vi "Dashboard Main.vi"() -> ()   [LabVIEW 2014]
uses:
  <vilib>/event_ctls.llb/eventvkey.ctl
  <vilib>/Rock Robotics/WPI/Dashboard/WPI_DashboardLogging Global.vi
  <vilib>/Rock Robotics/Network Tables/SD Read Number.vi
  <vilib>/Utility/config.llb/Write Key (String).vi
  <vilib>/Utility/config.llb/Write Key (I32).vi
  <vilib>/Rock Robotics/Network Tables/SD Write Numeric Array.vi
  <vilib>/Utility/config.llb/NI_LVConfig.lvlib
panel:
  out "Numeric":u32
  in  "TCP":refnum<k5>
  in  "Rec Mode":enum32{"Stop", "Record", "Playback"}(radio)
  in  "Vision":u16(ring) items=["Camera Off", "USB Camera SW", "USB Camera HW", "IP Camera"]
  in  "Dashboard Tab":T1(tab)
  in  "Camera Settings":T2={"Frame Rate"=30, "Compression"=30, "Size"=1} {"Frame Rate" scale=1.0..30.0; "Size" items=["640x480", "320x240", "160x120"]}
  out "Mode":T3(ring)=enum."Auto Disabled"
  in  "DB Camera Config":bool
  out "fps":dbl format="%#.1g"
  out "Mbps":dbl format="%#.1g"
  out "Mbps 2":bool
  out "Gyro":dbl(knob) scale=0.0..360.0
  out "Distance from Object":dbl(knob) scale=0.1..100.0
  out "Arm":dbl(slide) max=6.0 scale=0.0..6.0 scale format="%.6g"
  out "Totes":u8(slide) scale=0.0..6.0
  out "JS1 Z":dbl(slide) scale=-1.0..1.0 scale format="%#_2e"
  out "JS1 Graph":cluster{"X":dbl, "Y":dbl}[](graph)
  out "JS1 Buttons":T4
  out "MotorChart R":cluster{"Numeric":dbl, "Numeric":dbl}(graph)
  out "Battery Meter":dbl(slide) scale=0.0..14.0 scale format="%#_2e"
  out "MotorChart L":T5(graph)
  out "Robot Position":cluster{"Y":dbl[], "Y":dbl[]}[](graph)
  out "JS2 Z":dbl(slide) scale=-1.0..1.0 scale format="%#_2e"
  out "JS2 Graph":cluster{"X":dbl, "Y":dbl}[](graph)
  out "JS2 Buttons":T4
  in  "DB/String 9":string
  in  "DB/String 8":string
  in  "DB/String 7":string
  in  "DB/String 6":string
  in  "DB/String 5":string
  in  "DB/String 4":string
  in  "DB/String 3":string
  in  "DB/String 2":string
  in  "DB/String 1":string
  in  "DB/String 0":string
  in  "DB/Slider 0":dbl(slide) scale=0.0..5.0
  in  "DB/Slider 1":dbl(slide) scale=0.0..5.0
  in  "DB/Slider 2":dbl(slide) scale=0.0..5.0
  in  "DB/Slider 3":dbl(slide) scale=0.0..5.0
  out "DB/LED 3":bool
  out "DB/LED 2":bool
  out "DB/LED 1":bool
  out "DB/LED 0":bool
  in  "DB/Button 3":bool
  in  "DB/Button 2":bool
  in  "DB/Button 1":bool
  in  "DB/Button 0":bool caption="New Name"
  in  "Preset Auton Routine":T6(ring)
  in  "Action":T7(ring)
  out "X/Y/a Output":dbl[][](array[numeric]) caption="X pos     Y pos    Angle    Action"
  in  "If an object is detected...":T8(ring)
  in  "Input":dbl[](array[numeric])
  in  "Index No.":u8
  in  "Add Keyframe":bool
  in  "Remove Keyframe":bool
  in  "Load Preset":bool
  in  "Test Slider":dbl(slide) scale=0.0..100.0 scale format="%#_3g"
  in  "On/Off":bool caption="Solenoid"
  in  "Test Name":u16(ring) items=["Select the test to run...", "Example Test", "-------------------------------", "List of tests is built in robot code.", "Replace with your own automated tests."]
  in  "Test Tree":string(tree)
  in  "Motor":cluster{"Value":dbl, "Enable":bool} {"Value" scale=-1.0..1.0 scale format="%#_3g"}
  out "Progress":T9 {"Test Progress" scale=0.0..100.0}
  in  "Rev/Fwd":cluster{"Forward":bool, "Reverse":bool}
  in  "Test Ring":u16(ring) items=["Monochrome", "Color"]
  in  "Listbox":i32(listbox)
  out "Tree":string(tree)
  out "Camera Image":T10(plugin-control)
  out "Boolean":bool
  out "Camera IP":string
  out "Image Message":string="Timeout in Camera Communications"
  # "Left"
  # "Right"
  # "Batt"
  # "312"
  # "NOTE: Set Angle to -1 if you don't\nwant to reposition after movement.\nAngle relative to starting angle\n(unless gryo is present)"
  # "0"
  # "324"
  # "Values measured in inches"
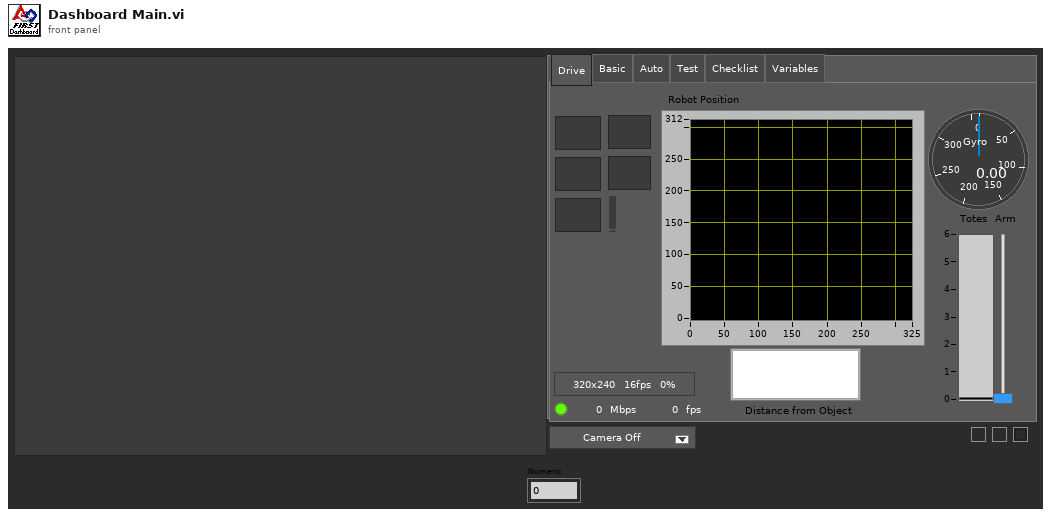
[diagram p1: front panel]
types:
  T1 = enum32{"Drive", "Basic", "Auto", "Test", "Checklist", "Variables"}
  T2 = cluster{"Frame Rate":i32, "Compression":i32, "Size":u16}
  T3 = enum8{"Tele-Op Disabled", "Tele-Op Enabled", "Auto Disabled", "Auto Enabled", "Test Disabled", "Test Enabled", "Disconnected", "No Code", "E-Stop"}
  T4 = cluster{bool, bool, bool, bool, bool, bool, bool, bool, bool, bool, bool, bool}
  T5 = cluster{"Numeric":dbl, "Numeric":dbl, "Battery V":dbl}
  T6 = enum8{"Score 3 Totes", "Move 1 Tote", "Score 3 Containers", "Move 1 Container", "Move 1 Tote & Container", "Get Center Step Containers", "Get Left Step Container", "Get Right Step Containter", "Custom..."}
  T7 = enum16{"Do Nothing", "Get Tote ", "Get Tote w/ Arms", "Get Container w/ Arms", "Stack Tote", "Place Object on Ground", "Eject Tote"}
  T8 = enum8{"Pick up (tote)", "Pick up (container)", "Avoid", "Wait until clear"}
  T9 = cluster{"Test Progress":u8, "Test Progress Text":string}
  T10 = typedef "IMAQ Image.ctl" = refnum<image>
  T11 = enum32{"Drive", "Basic", "Custom", "Test", "Checklist", "Variables"}
  T12 = typedef "Image Type" = u32
  T13 = cluster{"Camera Image":refnum<vi>, "Dashboard Tab":refnum<vi>, "Boolean":refnum<vi>, "Vision":refnum<vi>, "Rec Mode":refnum<vi>, "Test Slider":refnum<vi>, "On/Off ":refnum<vi>, "Test Ring":refnum<vi>, "Rev/Fwd":refnum<vi>, "Test Name":refnum<vi>, "Motor":refnum<vi>, "Progress":refnum<vi>, "CheckList":refnum<vi>, "Tree":refnum<vi>, "Test Tree":refnum<vi>}
  T14 = cluster{"Error Strings":string, "Disable Counts":cluster{u16, u16}, "Rail Faults":cluster{u16, u16, u16}, "Robot IP":string, "DB Mode":u8, "Event Info":cluster{"Name":string, "Type":u8, "Number":u16, "Replay":u8}, "Camera Addr":string}
  T15 = cluster{"Storage":cluster{"Disk Free":u64, "RAM Block":u32, "RAM free":u32}, "CPU Utilization":cluster{"CPU % ISR":sgl, "CPU % Time Crit":sgl, "CPU % Timed Str":sgl, "CPU % High":sgl, "CPU % Above":sgl, "CPU % Normal":sgl, "CPU % Low":sgl}, "CAN":cluster{"% Bus Utilization":sgl, "Bus Off Cnt":u32, "TX_FIFO Full Cnt":u32, "Receive Error Cnt":u8, "Transmit Error Cnt":u8}, "HID":cluster{"HID Outputs":u32, "Rumble Low":u16, "Rumble High":u16}[]}
  T16 = cluster{"Status bits":cluster{"Test Mode":bool, "Autonomous":bool, "Enabled":bool, "Code Start":bool, "Brownout":bool, "Reserved 2":bool, "Reserved 3":bool, "E-Stop":bool}, "Code Trace":cluster{"Disabled":bool, "TeleOp":bool, "Auto":bool, "Test":bool}, "Controller Type":enum16{"unknown", "cRIO", "roboRio"}, "Code?":enum16{"unknown", "noCode", "code"}, "Battery V":dbl}
  T17 = cluster{"Control Bits":cluster{"TestMode":bool, "Autonomous":bool, "Enabled":bool, "FMS Present":bool, bool, bool, bool, "E-Stop":bool}, "Team Station ":u8, "Countdown":sgl, "Joystick Values":cluster{"Axes":dbl[], "Buttons":bool[], "POVs":i16[]}[]}
  T18 = cluster{"Axes":dbl[], "Buttons":bool[], "POVs":i16[]}[]
  T19 = cluster{"[0]":i16, "[1]":i16, "[2]":i16, "[3]":i16, "[4]":i16, "[5]":i16, "[6]":i16, "[7]":i16, "[8]":i16}
  T20 = cluster{"Axes":dbl[], "Buttons":bool[], "POVs":i16[]}
  T21 = cluster{"Buttons[0]":bool, "Buttons[1]":bool, "Buttons[2]":bool, "Buttons[3]":bool, "Buttons[4]":bool, "Buttons[5]":bool, "Buttons[6]":bool, "Buttons[7]":bool, "Buttons[8]":bool, "Buttons[9]":bool, "Buttons[10]":bool, "Buttons[11]":bool}
  T22 = typedef "NI_LVConfig.lvlib/Config Data RefNum.ctl" = refnum<k1>
  T23 = cluster{"Operation":enum16{"Update", "Clear"}, "Color Box":u32}[]
  T24 = typedef "eventvkey.ctl" = enum16{"ASCII", "Enter", "Return", "Shift", "Ctrl", "Alt", "Cmd", "Opt", "Caps", "NumLock", "Clear", "Break", "Up", "Down", "Left", "Right", "Insert", "Delete", "Home", "End", "PageUp", "PageDown", "Escape", "Help", "Pause", "ScrollLock", "F1", "F2", "F3", "F4", "F5", "F6", "F7", "F8", "F9", "F10", "F11", "F12", "F13", "F14", "F15", "F16", "F17", "F18", "F19", "F20", "F21", "F22", "F23", "F24", "Play", "VolumeUp", "VolumeDown", "Mute", "Two Byte Char"}
  T25 = cluster{"Image Size":bool, "Image Type":bool, "Pixel Value":bool, "ROI Information":bool, "Zoom Factor":bool}
  T26 = enum8{"Enabled", "Disabled", "Disabled and Grayed Out"}
  T27 = cluster{"Operation":enum16{"Update", "Clear"}, "Color Box":u32}
  T28 = cluster{"Add Keyframe":bool, "Remove Keyframe":bool, "Load Preset":bool}
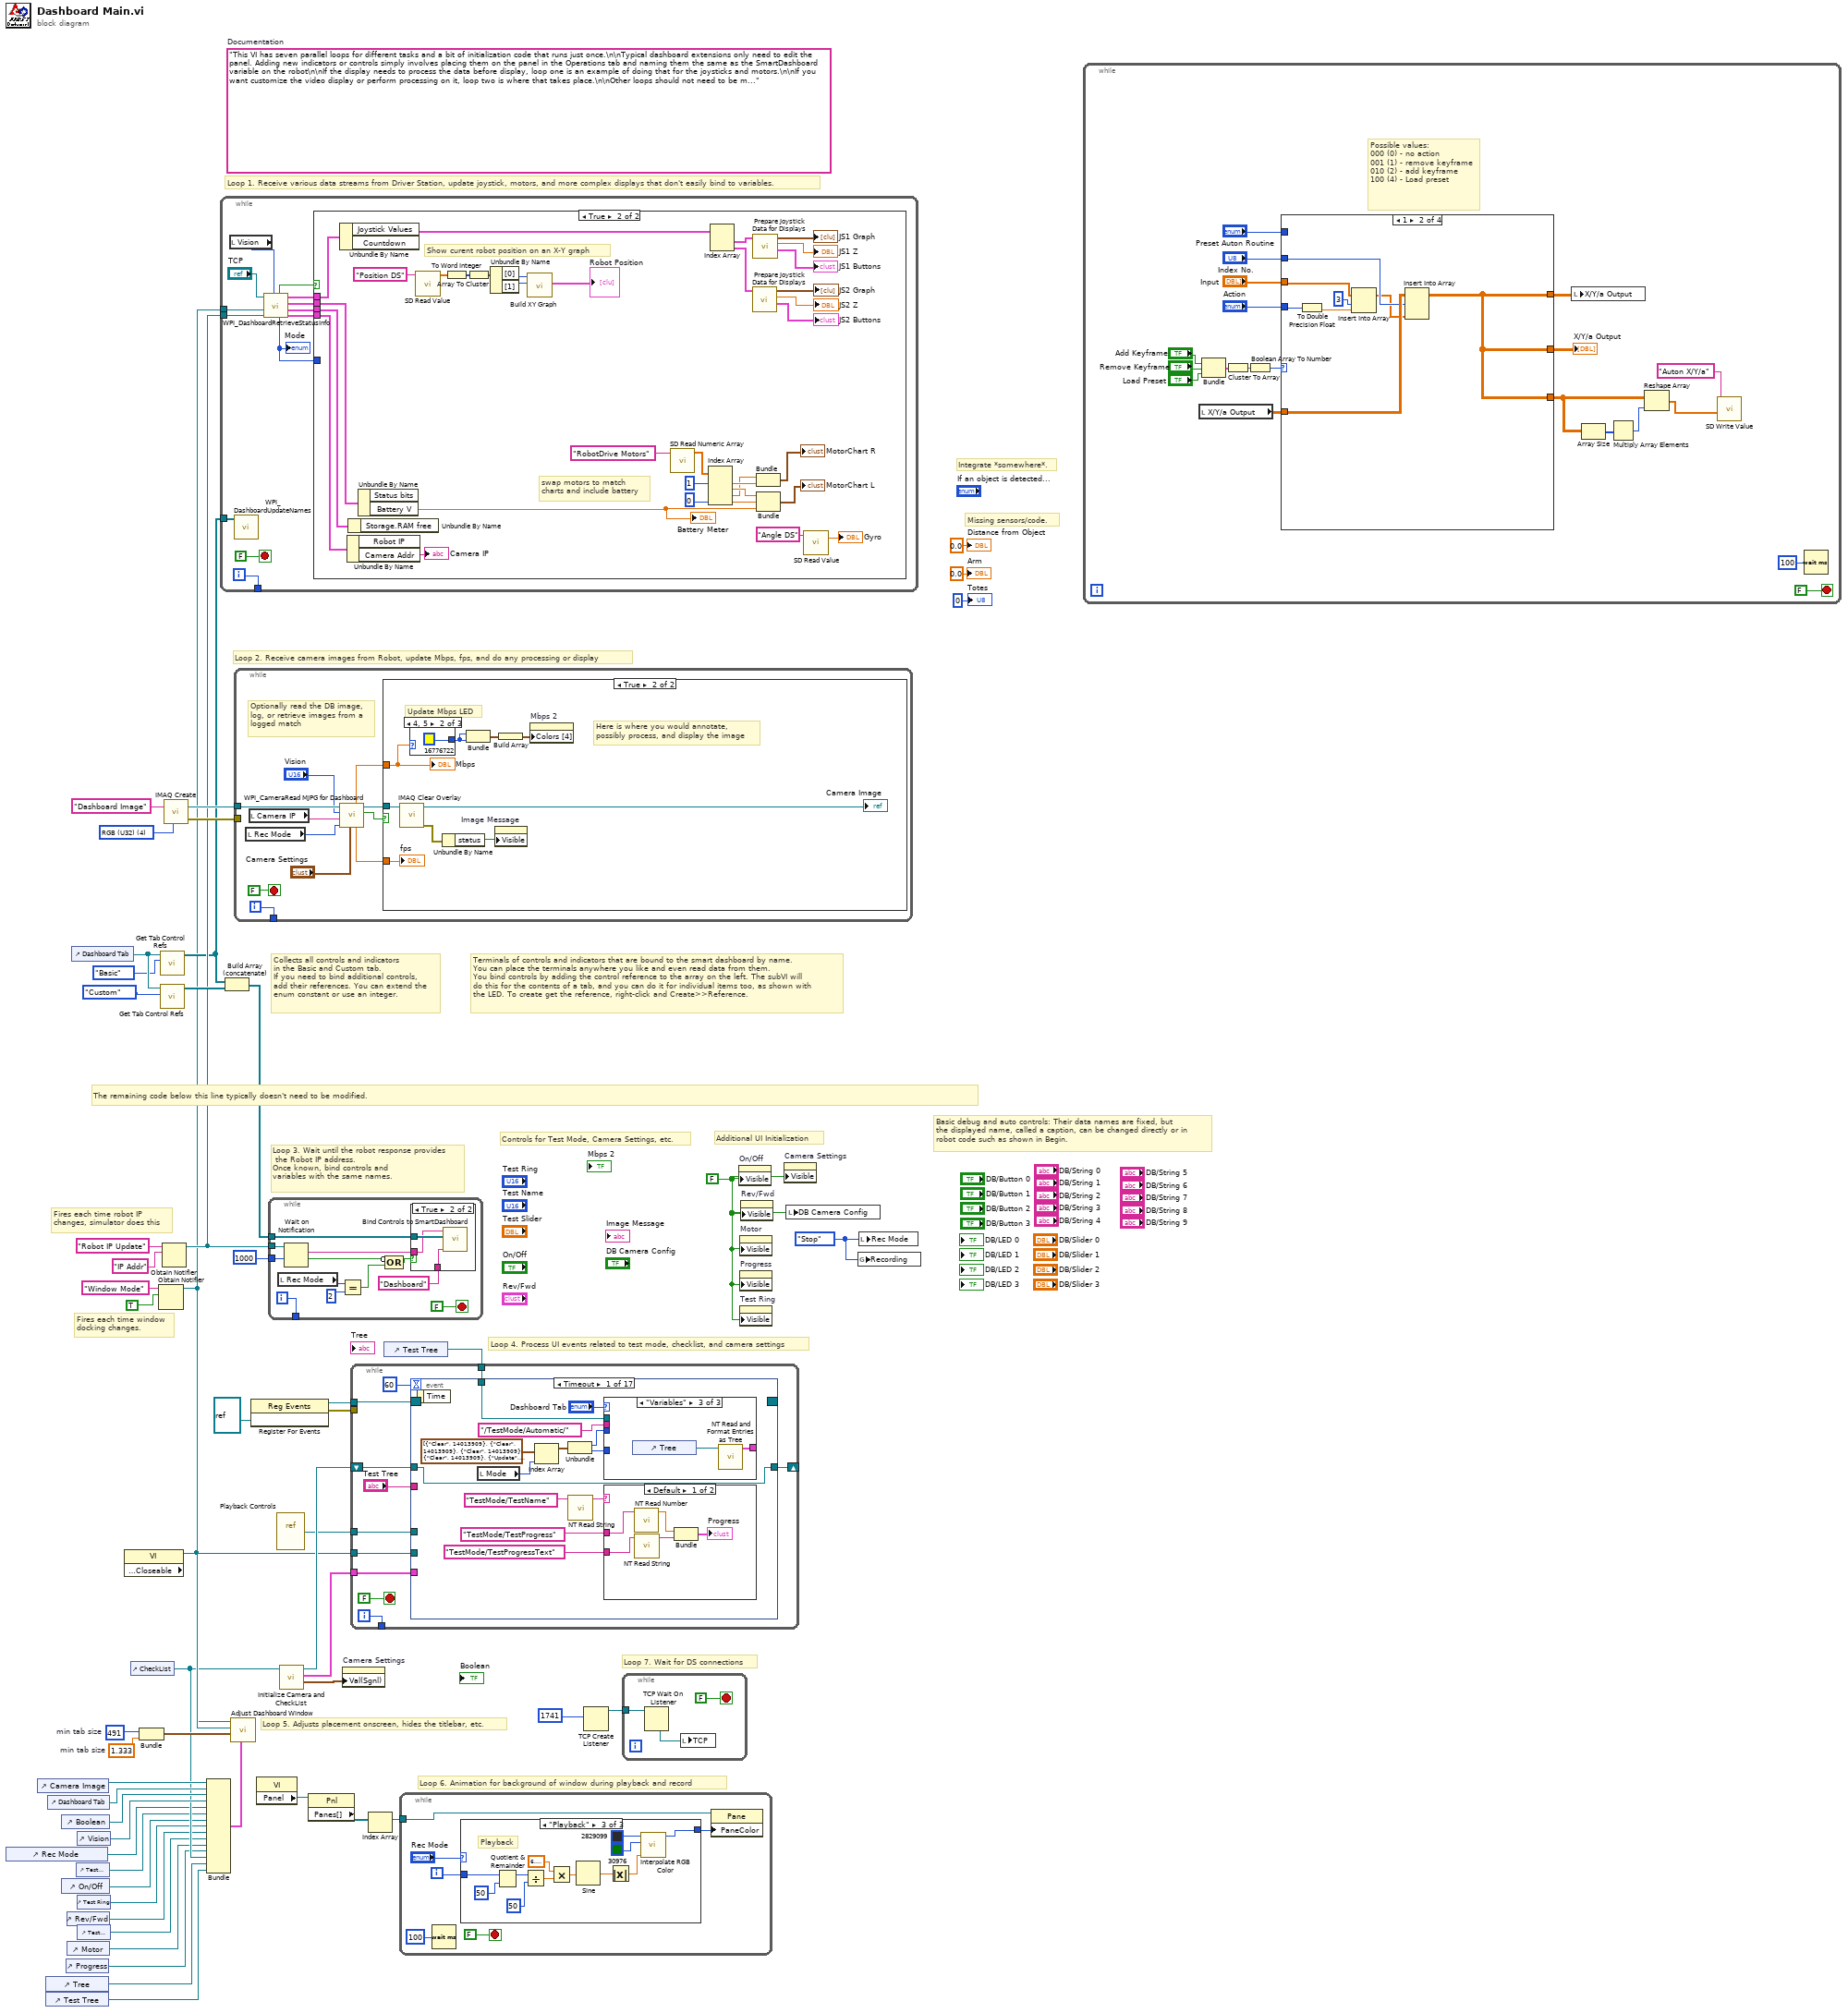
[diagram p0: block diagram]
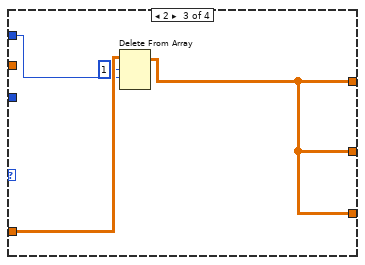
[diagram p3: hidden frame]
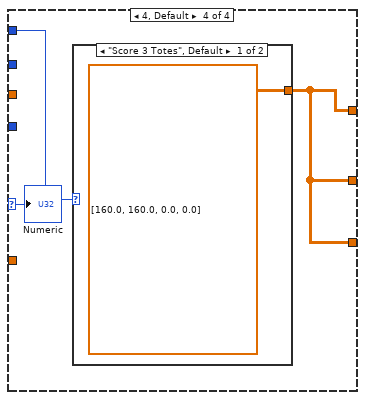
[diagram p4: hidden frame]
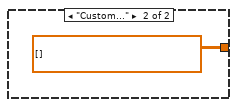
[diagram p5: hidden frame]
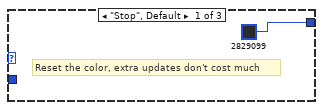
[diagram p7: hidden frame]
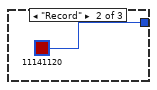
[diagram p8: hidden frame]
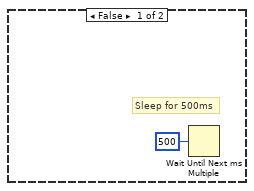
[diagram p10: hidden frame]
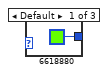
[diagram p11: hidden frame]
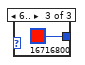
[diagram p12: hidden frame]
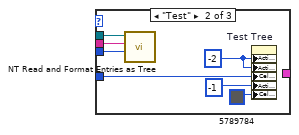
[diagram p14: hidden frame]
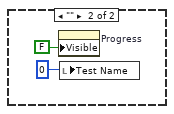
[diagram p15: hidden frame]
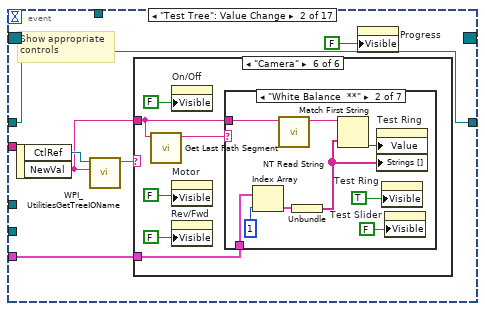
[diagram p16: hidden frame]
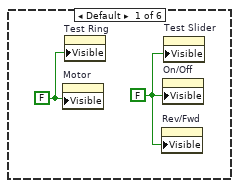
[diagram p17: hidden frame]
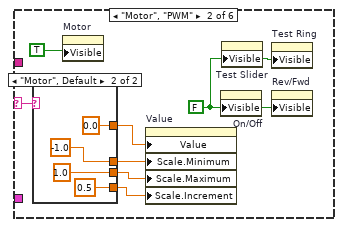
[diagram p18: hidden frame]
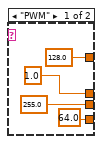
[diagram p19: hidden frame]
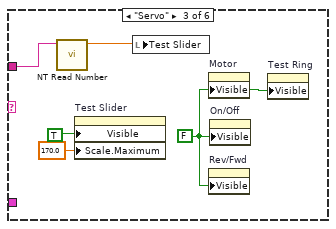
[diagram p20: hidden frame]
diagram:
  w27 = 491  # min tab size
  w26 = 1.333  # min tab size
  w35 = enum32{"Stop", "Record", "Playback"}."Stop" ("Rec Mode")
  w9 = FALSE ("Visible")
  (unwired) "This VI has seven parallel loops for different tasks and a bit of initialization code that runs just once.\n\nTypical dashboard extensions only need to edit the panel. Adding new indicators or controls simply involves placing them on the panel in the Operations tab and naming them the same as the SmartDashboard variable on the robot\n\nIf the display needs to process the data before display, loop one is an example of doing that for the joysticks and motors.\n\nIf you want customize the video display or perform processing on it, loop two is where that takes place.\n\nOther loops should not need to be modified. They are pretty standard, and document the task they perform."  # Documentation
  w55 = T12 4 items=["Grayscale (U8)", "Grayscale (I16)", "Grayscale (SGL)", "Complex (CSG)", "RGB (U32)", "HSL (U32)", "RGB (U64)"] ("Image Type")
  # "Integrate *somewhere*."
  # "Missing sensors/code."
  # "Loop 7. Wait for DS connections"
  # "Basic debug and auto controls: Their data names are fixed, but\nthe displayed name, called a caption, can be changed directly or in\nrobot code such as shown in Begin."
  # "Controls for Test Mode, Camera Settings, etc."
  # "Additional UI Initialization"
  # "Loop 6. Animation for background of window during playback and record"
  # "Fires each time robot IP\nchanges, simulator does this"
  # "Fires each time window\ndocking changes."
  # "Collects all controls and indicators\nin the Basic and Custom tab.\nIf you need to bind additional controls,\nadd their references. You can extend the\nenum constant or use an integer."
  # "The remaining code below this line typically doesn't need to be modified."
  # "Loop 4. Process UI events related to test mode, checklist, and camera settings"
  # "Terminals of controls and indicators that are bound to the smart dashboard by name.\nYou can place the terminals anywhere you like and even read data from them.\nYou bind controls by adding the control reference to the array on the left. The subVI will\ndo this for the contents of a tab, and you can do it for individual items too, as shown with\nthe LED. To create get the reference, right-click and Create>>Reference."
  # "Loop 3. Wait until the robot response provides\n the Robot IP address.\nOnce known, bind controls and\nvariables with the same names."
  # "Loop 5. Adjusts placement onscreen, hides the titlebar, etc."
  # "Loop 1. Receive various data streams from Driver Station, update joystick, motors, and more complex displays that don't easily bind to variables."
  # "Loop 2. Receive camera images from Robot, update Mbps, fps, and do any processing or display"
  n1 = control-ref of="Rec Mode"() -> (w15:refnum<vi>)
  n2 = control-ref of="Camera Image"() -> (w30:refnum<vi>)
  n3 = control-ref of="Tree"() -> (w19:refnum<vi>)
  n4 = control-ref of="Test Tree"() -> (w18:refnum<vi>)
  n5 = control-ref of="Dashboard Tab"() -> (w29:refnum<vi>)
  n6 = control-ref of="Boolean"() -> (w24:refnum<vi>)
  n7 = control-ref of="On/Off"() -> (w13:refnum<vi>)
  n8 = control-ref of="Progress"() -> (w10:refnum<vi>)
  n9 = control-ref of="Rev/Fwd"() -> (w11:refnum<vi>)
  n10 = control-ref of="Motor"() -> (w16:refnum<vi>)
  n11 = control-ref of="Dashboard Tab"() -> (w33:refnum<vi>)
  n12 = control-ref of="Test Slider"() -> (w14:refnum<vi>)
  n13 = control-ref of="Vision"() -> (w28:refnum<vi>)
  n14 = control-ref of="Test Ring"() -> (w12:refnum<vi>)
  n15 = control-ref of="Test Name"() -> (w17:refnum<vi>)
  n16 = property class="VI" props=["Front Panel.Closeable"]() -> (reference out=w34:refnum<vi>)  [unwired: 2 in, 2 out]
  n17 = control-ref of="CheckList"() -> (w20:refnum<vi>)
  n18 = Bundle("min tab size"=w27, "min tab size"=w26) -> (w25:cluster{"min tab size":i32, "min tab size":dbl})  [unwired: 1 in]
  n19 = Obtain Notifier(name (unnamed)="Window Mode", notification data type=TRUE) -> (notifier out=w6:refnum<notifier>)  [unwired: 2 in, 2 out]
  n20 = call <vilib>:"Get Tab Control Refs.vi"("Page Index"=T11."Basic" ("Dashboard Tab"), "TabControl in"=w33) -> ("ControlsOnPage"=w7:refnum<vi>[])  [unwired: 9 in]
  n21 = call <vilib>:"Get Tab Control Refs.vi"("Page Index"=T11."Custom" ("Dashboard Tab"), "TabControl in"=w33) -> ("ControlsOnPage"=w32:refnum<vi>[])  [unwired: 9 in]
  n22 = Obtain Notifier(name (unnamed)="Robot IP Update", notification data type="IP Addr" ("name (unnamed)")) -> (notifier out=w8:refnum<notifier>)  [unwired: 2 in, 2 out]
  n23 = call "IMAQ Create"("Image Name"="Dashboard Image", "Image Type"=w55) -> ("New Image"=w53:T10, "error out"=w52:errorcluster)  [unwired: 2 in, 1 out]
  n24 = Bundle("Camera Image"=w30, "Dashboard Tab"=w29, "Boolean"=w24, "Vision"=w28, "Rec Mode"=w15, "Test Slider"=w14, "On/Off"=w13, "Test Ring"=w12, "Rev/Fwd"=w11, "Test Name"=w17, "Motor"=w16, "Progress"=w10, "CheckList"=w20, "Tree"=w19, "Test Tree"=w18) -> (w21:T13)  [unwired: 1 in]
  n25 = while {
    tunnel: [w67] -> _
    tunnel: w8 -> [w61]
    tunnel: w7 -> [w60]
    tunnel: w6 -> [w56]
    i -> [w67]
    stop <- FALSE stop-if-true
    n26 = local read "Vision"() -> (w58:u16)
    n27 = call <vilib>:"WPI_DashboardUpdateNames.vi"("Controls on Tab"=w60) -> ()  [unwired: 11 in]
    n28 = call <vilib>:"WPI_DashboardRetrieveStatusInfo.vi"("Vision"=w58, "Binding Refnum"=w61, "Window Mode Notifier"=w56, "TCP Cnx"="TCP") -> ("Power and Errors"=w62:T14, "Robot Metrics"=w65:T15, "Status Info"=w66:T16, "Control Info"=w63:T17, "Robot Mode"=w59:T3, "Process?"=w64:bool)  [unwired: 2 in]
    "Mode" <- w59
    n29 = case shown="True" w64 {
      tunnel: w66 -> [_ w102]
      tunnel: w65 -> [_ w101]
      tunnel: w63 -> [_ w100]
      tunnel: w62 -> [_ w99]
      tunnel: w59 -> [_ _]
      frame False {
      }
      frame True {
        # "Show curent robot position on an X-Y graph"
        # "swap motors to match\ncharts and include battery"
        n30 = Unbundle By Name(w100) -> ("Joystick Values"=w88:T18)  [unwired: 1 out]
        n31 = Unbundle By Name(w99) -> ("Camera Addr"=→"Camera IP":string)  [unwired: 1 out]
        n32 = Unbundle By Name(w101) -> ()  [unwired: 1 out]
        n33 = Unbundle By Name(w102) -> ("Battery V"=w69:dbl)  [unwired: 1 out]
        "Battery Meter" <- w69
        n34 = call-poly <vilib>:"SD Read Value.vi"("Name"="Position DS") -> ("Numeric Array"=w74:dbl[])  [unwired: 8 in, 2 out]
        n35 = To Word Integer(number=w74) -> (16bit integer=w73:i16[])
        n36 = Array To Cluster(array=w73) -> (cluster=w72:T19)
        n37 = Unbundle By Name(w72) -> ("[0]"=w71:i16, "[1]"=w70:i16)
        n38 = call "Build XY Graph"("Y Input"=w70, "X Input"=w71) -> ("XY Graph"=→"Robot Position":cluster{"X":dbl[], "Y":dbl[]}[])  [unwired: 8 in, 1 out]
        n39 = call <vilib>:"SD Read Numeric Array.vi"("Name"="RobotDrive Motors") -> ("Numeric Array"=w90:dbl[])  [unwired: 8 in, 2 out]
        n40 = Index Array(array=w90, index #1=1, index #4=0) -> (element #1=w94:dbl, element #2=w95:dbl, element #3=w93:dbl, element #4=w98:dbl)  [unwired: 2 in]
        n41 = Index Array(array=w88) -> (element #1=w87:T20, element #2=w82:T20)  [unwired: 2 in]
        n42 = call "Prepare Joystick Data for Displays.vi"("Joystick Values"=w82) -> ("Buttons"=→"JS2 Buttons":T21, "Z Axis"=→"JS2 Z":dbl, "Cartesian Data"=→"JS2 Graph":cluster{"X axis":dbl, "X axis":dbl}[])  [unwired: 8 in]
        n43 = call "Prepare Joystick Data for Displays.vi"("Joystick Values"=w87) -> ("Buttons"=→"JS1 Buttons":T21, "Z Axis"=→"JS1 Z":dbl, "Cartesian Data"=→"JS1 Graph":cluster{"X axis":dbl, "X axis":dbl}[])  [unwired: 8 in]
        n44 = Bundle("Numeric"=w93, "Numeric"=w94) -> (→"MotorChart R":cluster{"Numeric":dbl, "Numeric":dbl})  [unwired: 1 in]
        n45 = Bundle("Numeric"=w95, "Numeric"=w98, "Battery V"=w69) -> (→"MotorChart L":T5)  [unwired: 1 in]
        n46 = call-poly <vilib>:"SD Read Value.vi"("Name"="Angle DS") -> ("Numeric"=→"Gyro":dbl)  [unwired: 8 in, 2 out]
      }
    }
  }
  n47 = Build Array (concatenate)(w7, w32) -> (w31:refnum<vi>[])
  n48 = call "Adjust Dashboard Window.vi"("Sizing Refnums"=w21, "Size Constraints"=w25, "VI"=w34, "Notifier in"=w6) -> ()  [unwired: 8 in]
  n49 = while {
    tunnel: w53 -> [w111]
    tunnel: w52 -> [_]
    tunnel: [w112] -> _
    i -> [w112]
    stop <- FALSE stop-if-true
    # "Optionally read the DB image,\nlog, or retrieve images from a\nlogged match"
    n50 = local read "Rec Mode"() -> (w105:enum32{"Stop", "Record", "Playback"})
    n51 = local read "Camera IP"() -> (w103:string)
    n52 = call <vilib>:"WPI_CameraRead MJPG for Dashboard.vi"("Camera Settings"="Camera Settings", "Rec Mode"=w105, "Camera IP"=w103, "Camera Mode"="Vision", "Refnum in"=w111) -> ("Active"=w109:bool, "Refnum out"=w110:T10, "FPS"=w108:dbl, "Bandwidth (Mbps)"=w107:dbl)  [unwired: 3 in]
    n53 = case shown="True" w109 {
      tunnel: w110 -> [_ w118]
      tunnel: w107 -> [_ w117]
      tunnel: w108 -> [_ w115]
      frame False {
        # "Sleep for 500ms"
        n54 = Wait Until Next ms Multiple(millisecond multiple=u32 500) -> ()  [unwired: 1 out]
      }
      frame True {
        # "Here is where you would annotate,\npossibly process, and display the image"
        # "Update Mbps LED"
        n55 = call "IMAQ Clear Overlay"("Image"=w118) -> ("error out"=w122:errorcluster, "Image Out"=→"Camera Image":T10)  [unwired: 2 in, 7 out]
        n56 = case shown="4, 5" w117 {
          tunnel: [u32 6618880 ("Color Box") u32 16776722 ("Color Box") u32 16716800 ("Color Box")] -> w119
          frame Default {
          }
          frame 4, 5 {
          }
          frame 6.. {
          }
        }
        n57 = Unbundle By Name(w122) -> ("status"=w123:bool)
        n58 = Bundle("Color Box"=w119, "Color Box"=w119) -> (w121:cluster{"Color Box":u32, "Color Box":u32})  [unwired: 1 out]
        n59 = property on="Image Message" class="Str"("Visible"=w123) -> ()  [unwired: 2 in, 2 out]
        n60 = Build Array(w121) -> (w120:cluster{"Color Box":u32, "Color Box":u32}[])
        n61 = property on="Mbps 2" class="Bool (strict)"("Colors [4]"=w120) -> ()  [unwired: 2 in, 2 out]
        "Mbps" <- w117
        "fps" <- w115
      }
    }
  }
  n62 = register-events(refnum<vi> refnum) -> (reference out=w39:refnum<event-registration>, error out=w38:errorcluster)  [unwired: 2 in]
  n63 = property class="VI"() -> ("Panel"=w42:refnum<vi>)  [unwired: 2 in, 2 out]
  n64 = while {
    tunnel: w31 -> [w138]
    tunnel: w8 -> [w136]
    tunnel: [w134] -> _
    tunnel: u32 1000 ("milliseconds to wait") -> [w133]
    i -> [w134]
    stop <- FALSE stop-if-true
    n65 = local read "Rec Mode"() -> (w129:enum32{"Stop", "Record", "Playback"})
    n66 = Wait on Notification(notifier=w136, timeout in ms (-1)=w133) -> (notification=w135:string, timed out?=w131:bool)  [unwired: 2 in, 2 out]
    n67 = Equal?(x=w129, y=u16 2 ("Rec Mode")) -> (x = y?=w130:bool)
    n68 = Compound Arithmetic op=OR(invert w131, w130) -> (w132:bool)
    n69 = case shown="True" w132 {
      tunnel: w138 -> [_ w141]
      tunnel: w135 -> [_ w140]
      tunnel: "Dashboard" -> [_ w139]
      frame False {
      }
      frame True {
        n70 = call <vilib>:"Bind Controls to SmartDashboard.vi"("Client Name"=w139, "Bound Control Refs"=w141, "Server IP Address"=w140) -> ()  [unwired: 9 in]
      }
    }
  }
  n71 = vi-ref "Playback Controls.vi"() -> (w40:refnum<vi>)
  n72 = call "Initialize Camera and CheckList.vi"("ListBox in"=w20) -> ("Cluster"=w46:cluster{"value":i32, "value":i32, "index":i32}, "Array"=w47:cluster{string[]}[], "File Refnum"=w45:T22)  [unwired: 8 in]
  n73 = property class="Pnl"(reference=w42) -> ("Panes[]"=w43:refnum<vi>[])  [unwired: 1 in, 2 out]
  n74 = property on="Camera Settings" class="Clust (strict)"("Val(Sgnl)"=w46) -> ()  [unwired: 2 in, 2 out]
  n75 = Index Array(array=w43) -> (element=w41:refnum<vi>)  [unwired: 1 in]
  n76 = control-ref of="Test Tree"() -> (w44:refnum<vi>)
  n77 = while {
    tunnel: w47 -> [w149]
    shift-right: [w148] -> _
    shift-left: w45 -> [w147]
    tunnel: [w146] -> _
    tunnel: w44 -> [w145]
    tunnel: w40 -> [w144]
    tunnel: w39 -> [w143]
    tunnel: w38 -> [_]
    tunnel: w34 -> [w142]
    i -> [w146]
    stop <- FALSE stop-if-true
    n78 = event shown="[0] Timeout" {
      selector: w143 -> [_ _ _ _ _ _ _ _ _ _ _ _ _ _ _ _ _]
      dyn-events: [_ _ _ _ _ _ _ _ _ _ _ _ _ w387 _ _ _] -> _
      timeout: u32 60 ("milliseconds to wait") -> [_ _ _ _ _ _ _ _ _ _ _ _ _ _ _ _ _]
      tunnel: w145 -> [w161 _ _ _ _ _ _ _ _ _ _ _ _ _ _ _ _]
      tunnel: "Test Tree" -> [_ _ _ _ _ _ _ _ w356 w364 w366 w370 w378 _ _ _ _]
      tunnel: w149 -> [_ w183 _ _ _ _ w320 w350 _ _ _ _ _ _ _ _ _]
      tunnel: [w157 w182 w281 w286 w294 w306 w319 w343 w355 w362 w365 w369 w377 w389 w403 w404 w414] -> w148
      tunnel: w147 -> [w157 w182 w281 w286 w294 w306 w318 w343 w355 w362 w365 w369 w377 w389 w403 w404 w414]
      tunnel: w144 -> [_ _ _ _ _ _ _ _ _ _ _ _ _ w390 _ w407 _]
      tunnel: w142 -> [_ _ _ _ _ _ _ _ _ _ _ _ _ w385 _ _ _]
      event Timeout {
        n79 = event-data() -> ()  [unwired: 1 in, 1 out]
        n80 = local read "Mode"() -> (w160:T3)
        n81 = Index Array(array=T23 [{"Operation"=enum."Clear", "Color Box"=14013909}, {"Operation"=enum."Clear", "Color Box"=14013909}, {"Operation"=enum."Clear", "Color Box"=14013909}, {"Operation"=enum."Clear", "Color Box"=14013909}, {"Operation"=enum."Update", "Color Box"=14013909}, {"Operation"=enum."Update", "Color Box"=16777215}, {"Operation"=enum."Clear", "Color Box"=14013909}, {"Operation"=enum."Clear", "Color Box"=14013909}, {"Operation"=enum."Clear", "Color Box"=14013909}], index=w160) -> (element=w155:T27)
        n82 = Unbundle(w155) -> ("Operation"=w154:enum16{"Update", "Clear"}, "Color Box"=w153:u32)
        n83 = call <vilib>:"NT Read String.vi"("Name"="TestMode/TestName") -> ("String"=w164:string)  [unwired: 9 in, 1 out]
        n84 = case shown="\"Variables\"" "Dashboard Tab" {
          tunnel: w161 -> [_ w172 _]
          tunnel: "/TestMode/Automatic/" ("Name Pattern") -> [_ w171 _]
          tunnel: w154 -> [_ w170 _]
          tunnel: [_ _ w174] -> _
          tunnel: w153 -> [_ w166 _]
          frame "Auto", Default {
          }
          frame "Test" {
            w169 = -2 ("Active Item:Row Number")
            n85 = call <vilib>:"NT Read and Format Entries as Tree.vi"("Operation"=w170, "Name Pattern"=w171, "Tree Refnum"=w172) -> ()  [unwired: 7 in, 2 out]
            n86 = property on="Test Tree" class="Tree (strict)"("Active Item Row Number"=w169, "ActiveColNum"=w169, "CellBG"=w166, "Active Item Row Number"=-1 ("Active Item:Row Number"), "CellBG"=u32 5789784 ("Color Box")) -> ()  [unwired: 2 in, 2 out]
          }
          frame "Variables" {
            n87 = control-ref of="Tree"() -> (w173:refnum<vi>)
            n88 = call <vilib>:"NT Read and Format Entries as Tree.vi"("Tree Refnum"=w173) -> ("Formatted Strings"=w174:cluster{"Name":string, "Value":string}[])  [unwired: 9 in, 1 out]
          }
        }
        n89 = case shown="Default" w164 {
          tunnel: "TestMode/TestProgress" ("Name") -> [w176 _]
          tunnel: "TestMode/TestProgressText" ("Name") -> [w175 _]
          frame Default {
            n90 = call <vilib>:"NT Read Number.vi"("Name"=w176) -> ("Numeric"=w177:dbl)  [unwired: 9 in, 1 out]
            n91 = call <vilib>:"NT Read String.vi"("Name"=w175) -> ("String"=w178:string)  [unwired: 9 in, 1 out]
            n92 = Bundle("Numeric"=w177, "String"=w178) -> (→"Progress":cluster{"Numeric":dbl, "String":string})  [unwired: 1 in]
          }
          frame "" {
            n93 = property on="Progress" class="Clust (strict)"("Visible"=FALSE) -> ()  [unwired: 2 in, 2 out]
            n94 = local write "Test Name"(u16 0) -> ()
          }
        }
      }
      event "Test Tree": Value Change {
        # "Show appropriate\ncontrols"
        n95 = event-data() -> ("CtlRef"=w186:refnum<vi>, "NewVal"=w184:string)  [unwired: 1 in]
        n96 = call <vilib>:"WPI_UtilitiesGetTreeIOName.vi"("NewVal"=w184, "TreeControl in"=w186) -> ("I/O Name"=w187:string)  [unwired: 9 in]
        n97 = case shown="\"Camera\"" w187 {
          selector: w187 -> [_ w194 _ w212 w221 _]
          tunnel: w184 -> [_ _ w209 w211 _ w228]
          tunnel: w183 -> [_ _ _ _ _ w227]
          frame Default {
            w189 = FALSE ("Visible")
            w188 = FALSE ("Visible")
            n98 = property on="Motor" class="Clust (strict)"("Visible"=w188) -> ()  [unwired: 2 in, 2 out]
            n99 = property on="Test Ring" class="Ring (strict)"("Visible"=w188) -> ()  [unwired: 2 in, 2 out]
            n100 = property on="Rev/Fwd" class="Clust (strict)"("Visible"=w189) -> ()  [unwired: 2 in, 2 out]
            n101 = property on="On/Off" class="Bool (strict)"("Visible"=w189) -> ()  [unwired: 2 in, 2 out]
            n102 = property on="Test Slider" class="Slide (strict)"("Visible"=w189) -> ()  [unwired: 2 in, 2 out]
          }
          frame "Motor", "PWM" {
            w195 = FALSE ("Visible")
            n103 = case shown="\"Motor\", Default" w194 {
              tunnel: [1.0 ("Value") -1.0 ("Value")] -> w193
              tunnel: [255.0 ("Value") 1.0 ("Value")] -> w192
              tunnel: [128.0 ("Value") 0.0 ("Value")] -> w191
              tunnel: [64.0 ("Value") 0.5 ("Value")] -> w190
              frame "PWM" {
              }
              frame "Motor", Default {
              }
            }
            n104 = property on="Motor" class="Clust (strict)"("Visible"=TRUE) -> ()  [unwired: 2 in, 2 out]
            n105 = property on="Value" class="Slide (strict)"("Value"=w191, "Scale.Minimum"=w193, "Scale.Maximum"=w192, "Scale.Increment"=w190) -> ()  [unwired: 2 in, 2 out]
            n106 = property on="On/Off" class="Bool (strict)"("Visible"=w195) -> ()  [unwired: 2 in, 2 out]
            n107 = property on="Test Slider" class="Slide (strict)"("Visible"=w195) -> ()  [unwired: 2 in, 2 out]
            n108 = property on="Test Ring" class="Ring (strict)"("Visible"=w195) -> ()  [unwired: 2 in, 2 out]
            n109 = property on="Rev/Fwd" class="Clust (strict)"("Visible"=w195) -> ()  [unwired: 2 in, 2 out]
          }
          frame "Servo" {
            w207 = FALSE ("Visible")
            n110 = call <vilib>:"NT Read Number.vi"("Name"=w209) -> ("Numeric"=w208:dbl)  [unwired: 9 in, 1 out]
            n111 = property on="Test Slider" class="Slide (strict)"("Visible"=TRUE, "Scale.Maximum"=170.0 ("Scale.Range:Maximum")) -> ()  [unwired: 2 in, 2 out]
            n112 = local write "Test Slider"(w208) -> ()
            n113 = property on="Motor" class="Clust (strict)"("Visible"=w207) -> ()  [unwired: 2 in, 2 out]
            n114 = property on="Rev/Fwd" class="Clust (strict)"("Visible"=w207) -> ()  [unwired: 2 in, 2 out]
            n115 = property on="On/Off" class="Bool (strict)"("Visible"=w207) -> ()  [unwired: 2 in, 2 out]
            n116 = property on="Test Ring" class="Ring (strict)"("Visible"=w207) -> ()  [unwired: 2 in, 2 out]
          }
          frame "Relay", "Solenoid" {
            w210 = FALSE ("Visible")
            n117 = property on="Motor" class="Clust (strict)"("Visible"=w210) -> ()  [unwired: 2 in, 2 out]
            n118 = property on="Test Slider" class="Slide (strict)"("Visible"=w210) -> ()  [unwired: 2 in, 2 out]
            n119 = Search and Replace String(input string=w211, search string="/Value  **", replace string="/Direction") -> (result string=w217:string)  [unwired: 5 in, 3 out]
            n120 = property on="Test Ring" class="Ring (strict)"("Visible"=w210) -> ()  [unwired: 2 in, 2 out]
            n121 = call <vilib>:"NT Read String.vi"("Name"=w217) -> ("String"=w215:string)  [unwired: 9 in, 1 out]
            n122 = Equal?(x="Both directions", y=w215) -> (x = y?=w213:bool)
            n123 = Not(x=w213) -> (.not. x?=w214:bool)
            n124 = property on="Rev/Fwd" class="Clust (strict)"("Visible"=w213) -> ()  [unwired: 2 in, 2 out]
            n125 = property on="On/Off" class="Bool (strict)"("Visible"=w214, "Caption.Text"=w212) -> ()  [unwired: 2 in, 2 out]
          }
          frame "Compressor", "Digital Out" {
            w220 = FALSE ("Visible")
            # "Get direction and finish"
            n126 = property on="Motor" class="Clust (strict)"("Visible"=w220) -> ()  [unwired: 2 in, 2 out]
            n127 = property on="Test Slider" class="Slide (strict)"("Visible"=w220) -> ()  [unwired: 2 in, 2 out]
            n128 = property on="Test Ring" class="Ring (strict)"("Visible"=w220) -> ()  [unwired: 2 in, 2 out]
            n129 = property on="On/Off" class="Bool (strict)"("Visible"=TRUE, "Caption.Text"=w221) -> ()  [unwired: 2 in, 2 out]
            n130 = property on="Rev/Fwd" class="Clust (strict)"("Visible"=FALSE) -> ()  [unwired: 2 in, 2 out]
          }
          frame "Camera" {
            n131 = call <vilib>:"Get Last Path Segment.vi"("String in"=w228) -> ("String out"=w229:string)  [unwired: 10 in]
            n132 = property on="On/Off" class="Bool (strict)"("Visible"=FALSE) -> ()  [unwired: 2 in, 2 out]
            n133 = property on="Motor" class="Clust (strict)"("Visible"=FALSE) -> ()  [unwired: 2 in, 2 out]
            n134 = property on="Rev/Fwd" class="Clust (strict)"("Visible"=FALSE) -> ()  [unwired: 2 in, 2 out]
            n135 = case shown="\"White Balance  **\"" w229 {
              tunnel: w228 -> [w235 w244 w253 w262 w271 _ w277]
              tunnel: w227 -> [w233 w241 w250 w259 w268 _ _]
              frame "Size  **" {
                n136 = Index Array(array=w233) -> (element=w232:cluster{string[]})  [unwired: 1 in]
                n137 = call <vilib>:"NT Read String.vi"("Name"=w235) -> ("String"=w234:string)  [unwired: 9 in, 1 out]
                n138 = Unbundle(w232) -> (w230:string[])
                n139 = Match First String(2:w230, 3:w234) -> (0:w231:i32)  [unwired: 1 out]
                n140 = property on="Test Ring" class="Ring (strict)"("Value"=w231, "Strings []"=w230) -> ()  [unwired: 2 in, 2 out]
                n141 = property on="Test Ring" class="Ring (strict)"("Visible"=TRUE) -> ()  [unwired: 2 in, 2 out]
                n142 = property on="Test Slider" class="Slide (strict)"("Visible"=FALSE) -> ()  [unwired: 2 in, 2 out]
              }
              frame "White Balance  **" {
                n143 = Index Array(array=w241, index=1) -> (element=w242:cluster{string[]})
                n144 = call <vilib>:"NT Read String.vi"("Name"=w244) -> ("String"=w243:string)  [unwired: 9 in, 1 out]
                n145 = Unbundle(w242) -> (w239:string[])
                n146 = Match First String(2:w239, 3:w243) -> (0:w238:i32)  [unwired: 1 out]
                n147 = property on="Test Ring" class="Ring (strict)"("Value"=w238, "Strings []"=w239) -> ()  [unwired: 2 in, 2 out]
                n148 = property on="Test Ring" class="Ring (strict)"("Visible"=TRUE) -> ()  [unwired: 2 in, 2 out]
                n149 = property on="Test Slider" class="Slide (strict)"("Visible"=FALSE) -> ()  [unwired: 2 in, 2 out]
              }
              frame "Exposure  **" {
                n150 = Index Array(array=w250, index=2) -> (element=w251:cluster{string[]})
                n151 = call <vilib>:"NT Read String.vi"("Name"=w253) -> ("String"=w252:string)  [unwired: 9 in, 1 out]
                n152 = Unbundle(w251) -> (w247:string[])
                n153 = Match First String(2:w247, 3:w252) -> (0:w248:i32)  [unwired: 1 out]
                n154 = property on="Test Ring" class="Ring (strict)"("Value"=w248, "Strings []"=w247) -> ()  [unwired: 2 in, 2 out]
                n155 = property on="Test Ring" class="Ring (strict)"("Visible"=TRUE) -> ()  [unwired: 2 in, 2 out]
                n156 = property on="Test Slider" class="Slide (strict)"("Visible"=FALSE) -> ()  [unwired: 2 in, 2 out]
              }
              frame "Exposure Priority  **" {
                n157 = Index Array(array=w259, index=3) -> (element=w260:cluster{string[]})
                n158 = call <vilib>:"NT Read String.vi"("Name"=w262) -> ("String"=w261:string)  [unwired: 9 in, 1 out]
                n159 = Unbundle(w260) -> (w256:string[])
                n160 = Match First String(2:w256, 3:w261) -> (0:w257:i32)  [unwired: 1 out]
                n161 = property on="Test Ring" class="Ring (strict)"("Value"=w257, "Strings []"=w256) -> ()  [unwired: 2 in, 2 out]
                n162 = property on="Test Ring" class="Ring (strict)"("Visible"=TRUE) -> ()  [unwired: 2 in, 2 out]
                n163 = property on="Test Slider" class="Slide (strict)"("Visible"=FALSE) -> ()  [unwired: 2 in, 2 out]
              }
              frame "Color Enable  **" {
                n164 = Index Array(array=w268, index=4) -> (element=w269:cluster{string[]})
                n165 = call <vilib>:"NT Read String.vi"("Name"=w271) -> ("String"=w270:string)  [unwired: 9 in, 1 out]
                n166 = Unbundle(w269) -> (w265:string[])
                n167 = Match First String(2:w265, 3:w270) -> (0:w266:i32)  [unwired: 1 out]
                n168 = property on="Test Ring" class="Ring (strict)"("Value"=w266, "Strings []"=w265) -> ()  [unwired: 2 in, 2 out]
                n169 = property on="Test Ring" class="Ring (strict)"("Visible"=TRUE) -> ()  [unwired: 2 in, 2 out]
                n170 = property on="Test Slider" class="Slide (strict)"("Visible"=FALSE) -> ()  [unwired: 2 in, 2 out]
              }
              frame Default {
                n171 = property on="Test Ring" class="Ring (strict)"("Visible"=FALSE) -> ()  [unwired: 2 in, 2 out]
                n172 = property on="Test Slider" class="Slide (strict)"("Visible"=FALSE) -> ()  [unwired: 2 in, 2 out]
              }
              frame "Brightness  **", "Color Level  **", "Compression  **", "FPS  **", "Sharpness  **" {
                n173 = call <vilib>:"NT Read Number.vi"("Name"=w277) -> ("Numeric"=w276:dbl)  [unwired: 9 in, 1 out]
                n174 = local write "Test Slider"(w276) -> ()
                n175 = property on="Test Slider" class="Slide (strict)"("Visible"=TRUE, "Scale.Maximum"=100.0 ("Scale.Range:Maximum")) -> ()  [unwired: 2 in, 2 out]
                n176 = property on="Test Ring" class="Ring (strict)"("Visible"=FALSE) -> ()  [unwired: 2 in, 2 out]
              }
            }
          }
        }
        n177 = property on="Progress" class="Clust (strict)"("Visible"=FALSE) -> ()  [unwired: 2 in, 2 out]
      }
      event "Test Name": Mouse Enter {
        # "Populate the ring with the list of tests"
        n178 = event-data() -> ()  [unwired: 1 in, 1 out]
        n179 = call <vilib>:"NT Read String Array.vi"("Name"="TestMode/TestList") -> ("String Array"=w285:string[])  [unwired: 9 in, 1 out]
        n180 = Build Array (concatenate)("Select the test to run...", w285) -> (w284:string[])
        n181 = property on="Test Name" class="Ring (strict)"("Strings []"=w284) -> ()  [unwired: 2 in, 2 out]
      }
      event "Test Name": Value Change {
        w287 = FALSE ("Visible")
        # "Tell the robot the test name to run"
        n182 = event-data() -> ("NewVal"=w291:u16)  [unwired: 1 in]
        n183 = property on="Test Name" class="Ring (strict)"() -> ("Strings []"=w292:string[])  [unwired: 2 in, 2 out]
        n184 = local write "Progress"(T9 {"Test Progress"=0, "Test Progress Text"=""} ("Progress")) -> ()
        n185 = Index Array(array=w292, index=w291) -> (element=w290:string)
        n186 = call <vilib>:"NT Write String.vi"("String"=w290, "Name"="TestMode/TestName") -> ()  [unwired: 9 in, 1 out]
        n187 = property on="Progress" class="Clust (strict)"("Visible"=TRUE) -> ()  [unwired: 2 in, 2 out]
        n188 = property on="Motor" class="Clust (strict)"("Visible"=w287) -> ()  [unwired: 2 in, 2 out]
        n189 = property on="Test Slider" class="Slide (strict)"("Visible"=w287) -> ()  [unwired: 2 in, 2 out]
        n190 = property on="On/Off" class="Bool (strict)"("Visible"=w287) -> ()  [unwired: 2 in, 2 out]
        n191 = property on="Rev/Fwd" class="Clust (strict)"("Visible"=w287) -> ()  [unwired: 2 in, 2 out]
        n192 = property on="Test Ring" class="Ring (strict)"("Visible"=w287) -> ()  [unwired: 2 in, 2 out]
      }
      event "Listbox": Double Click {
        # "Shift clears all"
        # "Update symbols on the listbox"
        n193 = event-data() -> ("PlatMods.Shift"=w295:bool, "Row"=w297:i32)  [unwired: 1 in]
        n194 = case shown="True" w295 {
          tunnel: w297 -> [w301 _]
          tunnel: 1 -> [w300 _]
          frame False {
            n195 = property on="Listbox" class="LstBox (strict)"() -> ("Item Symbols"=w299:i32[])  [unwired: 2 in, 2 out]
            n196 = Replace Array Subset(array=w299, new element=w300, index=w301) -> (w298:i32[])
            n197 = property on="Listbox" class="LstBox (strict)"("Item Symbols"=w298) -> ()  [unwired: 2 in, 2 out]
          }
          frame True {
            w302 = 0 ("Top Row")
            n198 = property on="Listbox" class="LstBox (strict)"() -> ("Number of Rows"=w304:u32)  [unwired: 2 in, 2 out]
            n199 = Initialize Array(0, w304) -> (w303:i32[])
            n200 = property on="Listbox" class="LstBox (strict)"("Top Row"=w302, "Value"=w302, "Item Symbols"=w303) -> ()  [unwired: 2 in, 2 out]
          }
        }
      }
      event "Listbox": Key Down {
        # "Update symbols on the listbox\nLeft and right keys check and uncheck"
        n201 = event-data() -> ("VKey"=w308:T24)  [unwired: 1 in]
        n202 = case shown="\"Left\", \"Right\"" w308 {
          selector: w308 -> [w313 _]
          tunnel: eventvkey."Left" ("VKey") -> [w311 _]
          frame "Left", "Right" {
            n203 = Equal?(x=w311, y=w313) -> (x = y?=w312:bool)
            n204 = Select(t=0, s=w312, f=1) -> (s? t:f=w314:i32)
            n205 = property on="Listbox" class="LstBox (strict)"() -> ("Item Symbols"=w317:i32[])  [unwired: 2 in, 2 out]
            n206 = Replace Array Subset(array=w317, new element=w314, index="Listbox") -> (w316:i32[])
            n207 = property on="Listbox" class="LstBox (strict)"("Item Symbols"=w316) -> ()  [unwired: 2 in, 2 out]
          }
          frame Default {
          }
        }
      }
      event "DB Camera Config": Value Change {
        # "Show or hide the cluster of controls, store in ini file"
        n208 = event-data() -> ("NewVal"=w321:bool)  [unwired: 1 in]
        n209 = case shown="False" w321 {
          tunnel: w320 -> [w330 _]
          tunnel: [w323 w341] -> w319
          tunnel: w318 -> [w322 w341]
          frame False {
            w337 = "Camera"
            w340 = FALSE ("Visible")
            n210 = local read "Camera Settings"() -> (w329:T2)
            n211 = Index Array(array=w330) -> (element=w333:cluster{string[]})  [unwired: 1 in]
            n212 = Unbundle(w329) -> ("Frame Rate"=w328:i32, "Compression"=w327:i32, "Size"=w331:u16)
            n213 = Unbundle(w333) -> (w332:string[])
            n214 = Index Array(array=w332, index=w331) -> (element=w326:string)
            n215 = call-poly <vilib>:"Write Key.vi"("section"=w337, "value"=w326, "key"="Size", "refnum"=w322) -> ("refnum out"=w339:T22)  [unwired: 2 in, 5 out]
            n216 = call-poly <vilib>:"Write Key.vi"("section"=w337, "value"=w328, "key"="FrameRate", "refnum"=w339) -> ("refnum out"=w338:T22)  [unwired: 1 in, 6 out]
            n217 = property on="Camera Settings" class="Clust (strict)"("Visible"=w340) -> ()  [unwired: 2 in, 2 out]
            n218 = local write "DB Camera Config"(w340) -> ()
            n219 = call-poly <vilib>:"Write Key.vi"("section"=w337, "value"=w327, "key"="Compression", "refnum"=w338) -> ("refnum out"=w324:T22)  [unwired: 1 in, 6 out]
            n220 = call <vilib>:"Close Config Data.vi"("refnum"=w324) -> ("file path"=w325:path)  [unwired: 2 in, 8 out]
            n221 = call <vilib>:"Open Config Data.vi"("configuration file path"=w325) -> ("refnum"=w323:T22)  [unwired: 8 in, 2 out]
          }
          frame True {
            n222 = property on="Camera Settings" class="Clust (strict)"("Visible"=TRUE) -> ()  [unwired: 2 in, 2 out]
          }
        }
      }
      event "Camera Settings": Value Change {
        # "Update summary string when any elements of DB camera change"
        n223 = event-data() -> ("NewVal"=w354:T2)  [unwired: 1 in]
        n224 = Index Array(array=w350) -> (element=w349:cluster{string[]})  [unwired: 1 in]
        n225 = Unbundle(w354) -> ("Frame Rate"=w345:i32, "Compression"=w344:i32, "Size"=w347:u16)
        n226 = Unbundle(w349) -> (w348:string[])
        n227 = Index Array(array=w348, index=w347) -> (element=w346:string)
        n228 = Format Into String(format string="%s   %dfps   %d%%", w346, w345, w344) -> (resulting string=w351:string)  [unwired: 2 in, 1 out]
        n229 = Build Array(w351) -> (w352:string[])
        n230 = property on="DB Camera Config" class="Bool (strict)"("Strings [4]"=w352) -> ()  [unwired: 2 in, 2 out]
      }
      event "Motor.Enable": Value Change {
        # "When the test mode otor enable helper is set, update that\ntree row item's value"
        n231 = event-data() -> ("NewVal"=w360:bool)  [unwired: 1 in]
        n232 = Unbundle("Motor") -> ("Value"=w359:dbl)  [unwired: 1 out]
        n233 = Select(t=w359, s=w360, f=0.0) -> (s? t:f=w357:dbl)
        n234 = call <vilib>:"NT Write Number.vi"("Numeric"=w357, "Name"=w356) -> ()  [unwired: 9 in, 1 out]
      }
      event "Test Slider": Value Change {
        # "When the test mode slider helper is set, update that\ntree row item's value"
        n235 = event-data() -> ("NewVal"=w363:dbl)  [unwired: 1 in]
        n236 = call <vilib>:"NT Write Number.vi"("Numeric"=w363, "Name"=w364) -> ()  [unwired: 9 in, 1 out]
      }
      event "On/Off": Value Change {
        # "When the test mode on/off helper value is set, update that\ntree row item's value"
        n237 = event-data() -> ("NewVal"=w368:bool)  [unwired: 1 in]
        n238 = Boolean To (0,1)(Boolean=w368) -> (0, 1=w367:i16)
        n239 = call <vilib>:"NT Write Number.vi"("Numeric"=w367, "Name"=w366) -> ()  [unwired: 9 in, 1 out]
      }
      event "Rev/Fwd": Value Change {
        # "When the test mode helper value for relays is set, update that\ntree row item's value"
        n240 = event-data() -> ("NewVal.Forward"=w376:bool, "NewVal.Reverse"=w375:bool)  [unwired: 1 in]
        n241 = Boolean To (0,1)(Boolean=w376) -> (0, 1=w372:i16)
        n242 = Boolean To (0,1)(Boolean=w375) -> (0, 1=w374:i16)
        n243 = Negate(x=w374) -> (-x=w373:i16)
        n244 = Add(x=w372, y=w373) -> (x+y=w371:i16)
        n245 = call <vilib>:"NT Write Number.vi"("Numeric"=w371, "Name"=w370) -> ()  [unwired: 9 in, 1 out]
      }
      event "Test Ring": Value Change {
        # "When a test mode helper value is selected from the ring,\nset the tree item's variable to the string value"
        n246 = event-data() -> ("NewVal"=w380:u16)  [unwired: 1 in]
        n247 = property on="Test Ring" class="Ring (strict)"() -> ("Strings []"=w381:string[])  [unwired: 2 in, 2 out]
        n248 = Index Array(array=w381, index=w380) -> (element=w379:string)
        n249 = call <vilib>:"NT Write String.vi"("String"=w379, "Name"=w378) -> ()  [unwired: 9 in, 1 out]
      }
      event "Rec Mode": Value Change {
        # "Update globals for recording mode and path to read log from.\nClear when logging and let NetworkTables set path for vision to\nuse."
        n250 = event-data() -> ("NewVal"=w391:enum32{"Stop", "Record", "Playback"})  [unwired: 1 in]
        n251 = global write "WPI_DashboardLogging Global.vi" "Logging Filename"(path "") -> ()
        n252 = case shown="\"Playback\"" w391 {
          tunnel: w390 -> [_ w393 w401]
          tunnel: [_ _ w400] -> w387
          tunnel: [_ _ w399] -> _
          tunnel: w385 -> [_ _ w397]
          tunnel: cluster{i32, i32} {-250, 170} -> [_ _ w396]
          tunnel: [_ _ T25 {"Image Size"=TRUE, "Image Type"=TRUE, "Pixel Value"=TRUE, "ROI Information"=TRUE, "Zoom Factor"=FALSE} ("Image Information Shown:All Elements")] -> w383
          tunnel: [_ _ TRUE ("Zoom Factor")] -> w382
          frame Default {
          }
          frame "Stop", "Record" {
            # "Place Window too"
            n253 = invoke class="VI" method="FP.Close"(reference=w393) -> (reference out=w392:refnum<vi>)  [unwired: 2 in, 2 out]
            n254 = invoke class="VI" method="Abort VI"(reference=w392) -> ()  [unwired: 2 in, 3 out]
          }
          frame "Playback" {
            n255 = call "Open Playback Panel.vi"("Offset"=w396, "DB VI Ref"=w397, "Playback in"=w401) -> ("Playback out"=w398:refnum<vi>)  [unwired: 8 in]
            n256 = register-events(w398) -> (reference out=w400:refnum<event-registration>, error out=w399:errorcluster)  [unwired: 2 in]
          }
        }
        n257 = global write "WPI_DashboardLogging Global.vi" "Recording"(w391) -> ()
        n258 = property on="Camera Image" class="ImageControl"("Image Information Shown"=w383, "Image Information Visible"=w382) -> ()  [unwired: 2 in, 2 out]
        n259 = call <vilib>:"WPI_DashboardNT Log FieldName Cache.vi"("Operation"=enum16{"Lookup/Add", "Index", "Clear"}."Clear") -> ()  [unwired: 8 in, 3 out]
      }
      event Panel Close {
        w402 = enum32{"Stop", "Record", "Playback"}."Stop" ("Rec Mode")
        # "Playback window has been closed, abort"
        n260 = event-data() -> ()  [unwired: 1 in, 4 out]
        n261 = local write "Rec Mode"(w402) -> ()
        n262 = global write "WPI_DashboardLogging Global.vi" "Recording"(w402) -> ()
      }
      event Panel Close {
        # "Abort playback window and ourself"
        n263 = event-data() -> ()  [unwired: 1 in, 4 out]
        n264 = invoke class="VI" method="FP.Close"(reference=w407) -> (reference out=w406:refnum<vi>)  [unwired: 2 in, 2 out]
        n265 = invoke class="VI" method="Abort VI"(reference=w406) -> (error out=w405:errorcluster)  [unwired: 2 in, 2 out]
        n266 = invoke class="VI" method="Abort VI"(error in=w405) -> ()  [unwired: 2 in, 3 out]
      }
      event "Vision": Value Change {
        # "Enable/Disable Compression slider.\nHW USB is hard-coded into the camera"
        n267 = event-data() -> ("NewVal"=w413:u16)  [unwired: 1 in]
        n268 = Equal?(x=w413, y=u32 2 ("milliseconds to wait")) -> (x = y?=w411:bool)
        n269 = Select(t=T26."Disabled and Grayed Out" ("Disabled"), s=w411, f=T26."Enabled" ("Disabled")) -> (s? t:f=w408:T26)
        n270 = property on="Compression" class="Slide (strict)"("DisabledEnum"=w408) -> ()  [unwired: 2 in, 2 out]
      }
    }
  }
  n271 = while {
    tunnel: w41 -> [w416]
    i -> [w419]
    stop <- FALSE stop-if-true
    n272 = Wait (ms)(milliseconds to wait=u32 100) -> ()  [unwired: 1 out]
    n273 = case shown="\"Playback\"" "Rec Mode" {
      tunnel: w419 -> [_ _ w434]
      tunnel: [u32 2829099 ("Base Color") u32 11141120 ("Target Color") w423] -> w415
      frame "Stop", Default {
        # "Reset the color, extra updates don't cost much"
      }
      frame "Record" {
      }
      frame "Playback" {
        # "Playback"
        n274 = Quotient & Remainder(x=w434, y=u32 50 ("milliseconds to wait")) -> (x-y*floor(x/y)=w430:u32)  [unwired: 1 out]
        n275 = Divide(x=w430, y=u32 50 ("milliseconds to wait")) -> (x/y=w427:dbl)
        n276 = Multiply(x=6.283185307179586, y=w427) -> (x*y=w432:dbl)
        n277 = Sine(x=w432) -> (sin(x)=w431:dbl)
        n278 = Absolute Value(x=w431) -> (abs(x)=w424:dbl)
        n279 = call "Interpolate RGB Color.vi"("Proportion"=w424, "Target Color"=u32 30976, "Base Color"=u32 2829099) -> ("Result Color"=w423:u32)  [unwired: 8 in]
      }
    }
    n280 = property class="Pane"(reference=w416, "PaneColor"=w415) -> ()  [unwired: 1 in, 2 out]
  }
  n281 = TCP Create Listener(10:u16 1741 ("timeout ms (25000)")) -> (3:w4:refnum<k5>)  [unwired: 4 in, 2 out]
  n282 = while {
    tunnel: w4 -> [w436]
    stop <- FALSE stop-if-true
    n283 = TCP Wait On Listener(11:w436) -> (4:w435:refnum<k5>)  [unwired: 3 in, 4 out]
    n284 = local write "TCP"(w435) -> ()
  }
  n285 = property on="On/Off" class="Bool (strict)"("Visible"=w9) -> ()  [unwired: 2 in, 2 out]
  n286 = property on="Motor" class="Clust (strict)"("Visible"=w9) -> ()  [unwired: 2 in, 2 out]
  n287 = property on="Progress" class="Clust (strict)"("Visible"=w9) -> ()  [unwired: 2 in, 2 out]
  n288 = property on="Test Ring" class="Ring (strict)"("Visible"=w9) -> ()  [unwired: 2 in, 2 out]
  n289 = property on="Rev/Fwd" class="Clust (strict)"("Visible"=w9) -> ()  [unwired: 2 in, 2 out]
  n290 = property on="Camera Settings" class="Clust (strict)"("Visible"=w9) -> ()  [unwired: 2 in, 2 out]
  n291 = local write "DB Camera Config"(w9) -> ()
  n292 = global write "WPI_DashboardLogging Global.vi" "Recording"(w35) -> ()
  n293 = local write "Rec Mode"(w35) -> ()
  n294 = while {
    stop <- FALSE stop-if-true
    # "Possible values:\n000 (0) - no action\n001 (1) - remove keyframe\n010 (2) - add keyframe\n100 (4) - Load preset"
    n295 = local read "X/Y/a Output"() -> (w447:dbl[][])
    n296 = Bundle("Add Keyframe"="Add Keyframe", "Remove Keyframe"="Remove Keyframe", "Load Preset"="Load Preset") -> (w455:T28)  [unwired: 1 in]
    n297 = Cluster To Array(cluster=w455) -> (array=w454:bool[])
    n298 = Boolean Array To Number(Boolean array=w454) -> (number=w453:u32)
    n299 = case shown="1" w453 {
      selector: w453 -> [_ _ _ w471]
      tunnel: "Index No." -> [_ w461 w469 _]
      tunnel: "Input" -> [_ w466 _ _]
      tunnel: "Action" -> [_ w463 _ _]
      tunnel: [w458 w459 w467 w472] -> w449
      tunnel: [w458 w459 w467 w472] -> w448
      tunnel: w447 -> [w458 w462 w470 _]
      tunnel: "Preset Auton Routine" -> [_ _ _ w473]
      tunnel: [w458 w459 w467 w472] -> w445
      frame 0 {
        # "[do nothing]"
      }
      frame 1 {
        n300 = To Double Precision Float(number=w463) -> (double precision float=w464:dbl)
        n301 = Insert Into Array(array=w466, index=3, new element=w464) -> (w460:dbl[])
        n302 = Insert Into Array(array=w462, index (row)=w461, new element=w460) -> (w459:dbl[][])  [unwired: 1 in]
      }
      frame 2 {
        n303 = Delete From Array(array=w470, length=1, index (row)=w469) -> (array with subset deleted=w467:dbl[][])  [unwired: 1 in, 1 out]
      }
      frame 4, Default {
        n304 = case shown="\"Score 3 Totes\", Default" w473 {
          tunnel: [dbl[][] [[160.0, 160.0, 0.0, 0.0]] dbl[][] []] -> w472
          frame "Score 3 Totes", Default {
          }
          frame "Custom..." {
          }
        }
        "Numeric" <- w471
      }
    }
    "X/Y/a Output" <- w449
    n305 = local write "X/Y/a Output"(w448) -> ()
    n306 = Array Size(array=w445) -> (size(s)=w444:i32[])
    n307 = Multiply Array Elements(1:w444) -> (0:w443:i32)
    n308 = Reshape Array(w445, w443) -> (w442:dbl[])
    n309 = call-poly <vilib>:"SD Write Value.vi"("Numeric Array"=w442, "Name"="Auton X/Y/a") -> ()  [unwired: 8 in, 2 out]
    n310 = Wait (ms)(milliseconds to wait=u32 100) -> ()  [unwired: 1 out]
  }
  "Distance from Object" <- 0.0 ("Distance from Object")
  "Arm" <- 0.0 ("Arm")
  "Totes" <- u8 0 ("Totes")
